vi "ActDriveThenBalance.vi"(9 "FirstTime":bool, 10 "MaxSpeed (ft/s)":dbl, 11 "Dist (ft)":dbl) -> (1 "XSpeedDemand":dbl, 3 "Done":bool)   [LabVIEW 2023]
doc: "Robot will set the \"GyroZero\"drive forward straight a set distance utilizing position control, and then will balance for remaining time this vi is called\n\nInputs:\n-- MaxSpeed -- Double -- in ft/s, the MaxSpeed the robot can go -- \n-- Dist (ft) -- Double -- Distance in feet you want the robot to go -- \n-- FirstTime -- Boolean -- Input true the first time this function is called, sets the target position -- \n\nOutputs:\n-- Done -- Bool -- has the robot reached its target distance\n-- LeftSpeedDemand -- Double -- Speed Demand for left drive train inorder to reach target -- \n-- RightSpeedDemand -- Double -- Speed Demand for left drive train inorder to reach target --"
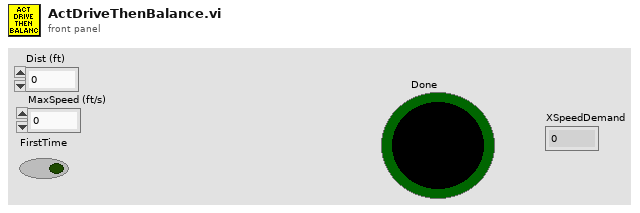
[diagram p1: front panel]
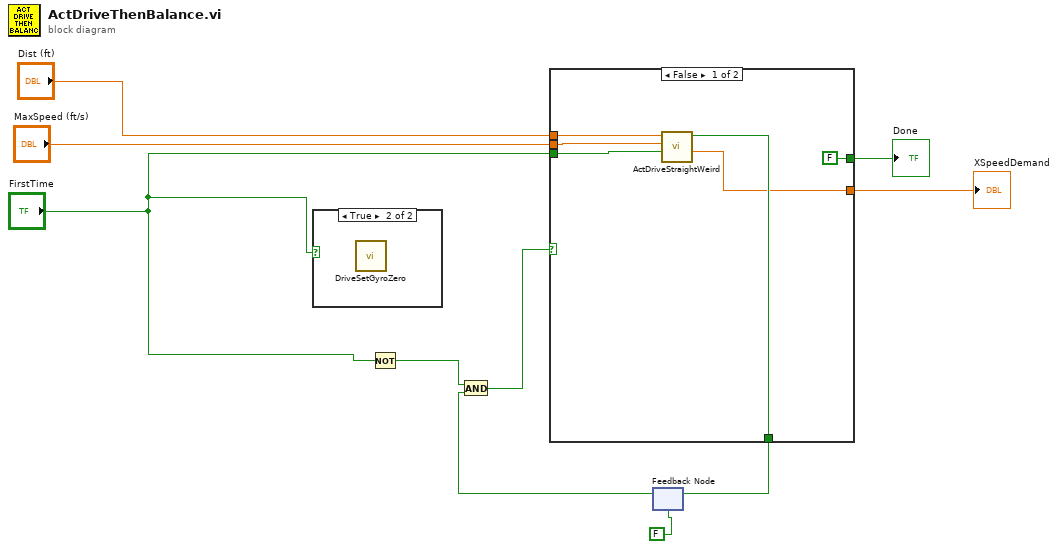
[diagram p0: block diagram]
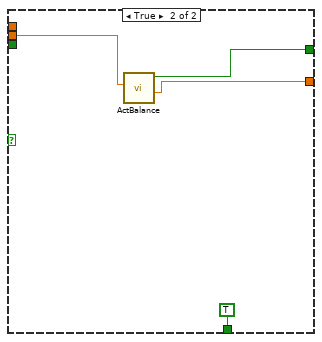
[diagram p3: hidden frame]
diagram:
  n1 = case shown="True" "FirstTime" {
    frame False {
    }
    frame True {
      n2 = call "DriveSetGyroZero.vi"() -> ()  [unwired: 11 in, 1 out]
    }
  }
  n3 = Not(x="FirstTime") -> (.not. x?=w2:bool)
  n4 = feedback #1(FALSE) -> (w3:bool)
  n5 = And(x=w2, y=w3) -> (x .and. y?=w4:bool)
  n6 = case shown="False" w4 {
    tunnel: "FirstTime" -> [w11 _]
    tunnel: "MaxSpeed (ft/s)" -> [w14 w20]
    tunnel: "Dist (ft)" -> [w15 _]
    tunnel: [w13 TRUE ("Done")] -> w5
    tunnel: [w12 w19] -> w8
    tunnel: [FALSE ("Done") w17] -> w7
    frame False {
      n7 = call "ActDriveStraightWeird.vi"("FirstTime"=w11, "MaxSpeed (ft/s)"=w14, "Dist (ft)"=w15) -> ("XSpeedDemand"=w12:dbl, "Done"=w13:bool)  [unwired: 7 in]
    }
    frame True {
      n8 = call "ActBalance.vi"("MaxSpeed (ft/s)"=w20) -> ("XSpeedDemand"=w19:dbl, "Done"=w17:bool)  [unwired: 9 in]
    }
  }
  "Done" <- w7
  "XSpeedDemand" <- w8
  n9 = feedback-in #1(w5) -> ()
